vi "set key length for variable length cipher.vi"(8 "error in":errorcluster, 10 "key length":i32, 11 "lvlibcrypto digest in":refnum<class "lvlibcrypto cipher.lvclass">) -> (0 "error out":errorcluster, 2 "key length out":i32, 3 "lvlibcrypto digest out":refnum<class "lvlibcrypto cipher.lvclass">)   [LabVIEW 2016, in "lvlibcrypto cipher.lvclass"]
doc: "EVP_rc4()\nRC4 stream cipher. This is a variable key length cipher with default key length 128 bits.\n \nEVP_rc2_cbc(), EVP_rc2_ecb(), EVP_rc2_cfb(), EVP_rc2_ofb()\nRC2 encryption algorithm in CBC, ECB, CFB and OFB modes respectively. This is a variable key length cipher with an additional parameter called \"effective key bits\" or \"effective key length\". By default both are set to 128 bits.\n \n \nEVP_rc2_40_cbc(), EVP_rc2_64_cbc()\nRC2 algorithm in CBC mode with a default key length and effective key length of 40 and 64 bits. These are obsolete and new code should use EVP_rc2_cbc(), EVP_CIPHER_CTX_set_key_length(), and EVP_CIPHER_CTX_ctrl() to set the key length and effective key length.\n \n \nEVP_bf_cbc(), EVP_bf_ecb(), EVP_bf_cfb(), EVP_bf_ofb()\nBlowfish encryption algorithm in CBC, ECB, CFB and OFB modes respectively. This is a variable key length cipher.\n \n \nEVP_cast5_cbc(), EVP_cast5_ecb(), EVP_cast5_cfb(), EVP_cast5_ofb()\nCAST encryption algorithm in CBC, ECB, CFB and OFB modes respectively. This is a variable key length cipher.\n \n \nEVP_rc5_32_12_16_cbc(), EVP_rc5_32_12_16_ecb(), EVP_rc5_32_12_16_cfb(), EVP_rc5_32_12_16_ofb()\nRC5 encryption algorithm in CBC, ECB, CFB and OFB modes respectively. This is a variable key length cipher with an additional \"number of rounds\" parameter. By default the key length is set to 128 bits and 12 rounds."
uses:
  lvlibcrypto cipher.lvclass
  lvlibcrypto cipher.lvclass/lvlibcrypto cipher.ctl
  lv tls dll.lvlib
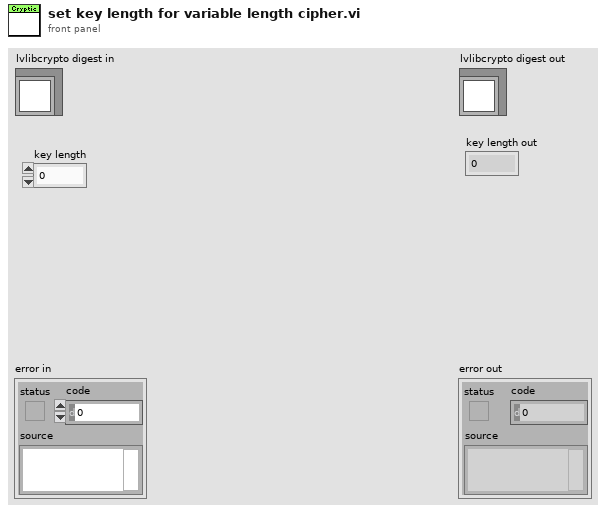
[diagram p1: front panel]
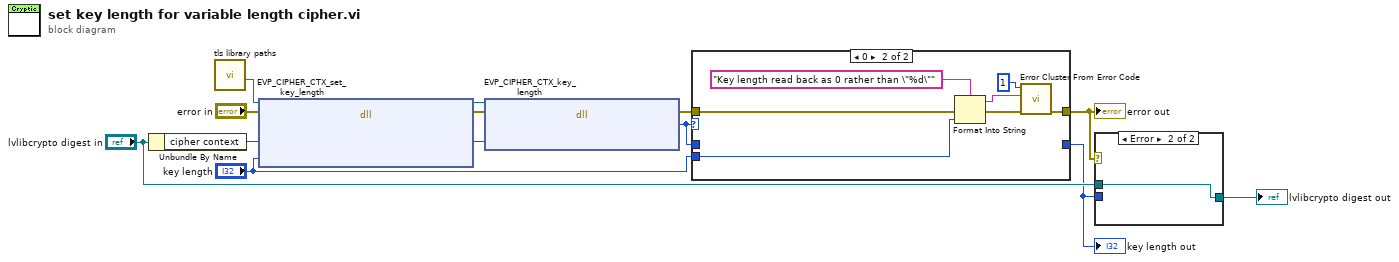
[diagram p0: block diagram]
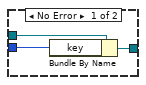
[diagram p2: hidden frame]
diagram:
  n1 = Unbundle By Name("lvlibcrypto digest in") -> ("cipher context"=w11:u64)
  n2 = call "tls library paths.vi"() -> ("libcrypto"=w13:path)  [unwired: 8 in, 3 out]
  n3 = dll-call lib="C:/Users/IEUser/Desktop/tlssimple/libcrypto-41.dll" fn="EVP_CIPHER_CTX_set_key_length"(path in=w13, error in="error in", "context"=w11, "key length"="key length") -> (path out=w8:path, error out=w10:errorcluster, "context"=w9:u64)  [unwired: 3 in]
  n4 = dll-call lib="C:/Users/IEUser/Desktop/tlssimple/libcrypto-41.dll" fn="EVP_CIPHER_CTX_key_length"(path in=w8, error in=w10, "context"=w9) -> (error out=w5:errorcluster, "size"=w3:i32)  [unwired: 2 in, 1 out]
  n5 = case shown="0" w3 {
    tunnel: [w15 w21] -> w1
    tunnel: w5 -> [w15 w22]
    tunnel: [w14 _] -> w4
    tunnel: w3 -> [w14 _]
    tunnel: "key length" -> [_ w16]
    frame Default {
    }
    frame 0 {
      n6 = Format Into String(format string="Key length read back as 0 rather than \"%d\"", error in=w22, w16) -> (resulting string=w18:string, error out=w19:errorcluster)  [unwired: 1 in]
      n7 = call <vilib>:"Error Cluster From Error Code.vi"("error in (no error)"=w19, "error message (\"\")"=w18, "error code (0)"=1) -> ("error out"=w21:errorcluster)  [unwired: 6 in]
    }
  }
  "error out" <- w1
  "key length out" <- w4
  n8 = case shown="Error" w1 {
    tunnel: "lvlibcrypto digest in" -> [w25 w26]
    tunnel: [w24 w26] -> w6
    tunnel: w4 -> [w23 _]
    frame No Error {
      n9 = Bundle By Name(cluster=w25, "key"=w23) -> (w24:refnum<class "lvlibcrypto cipher.lvclass">)
    }
    frame Error {
    }
  }
  "lvlibcrypto digest out" <- w6
